vi "1-Integer Parity Detector.vi"() -> ()   [LabVIEW 2014]
panel:
  out "Odd?":bool
  in  "Integer Picker":i32
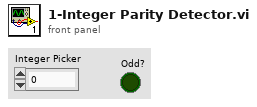
[diagram p1: front panel]
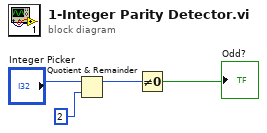
[diagram p0: block diagram]
diagram:
  n1 = Quotient & Remainder(x="Integer Picker", y=2) -> (x-y*floor(x/y)=w2:i32)  [unwired: 1 out]
  n2 = Not Equal To 0?(x=w2) -> (x != 0?=→"Odd?":bool)
